vi "Hide not selected Sub-Ctls.vi"(6 "sub":T1[](array[typedef]), 8 "error in":errorcluster, 9 "Sub-Ctls":refnum<vi>[](array[refnum]), 10 "Sub-Ctl Visible":refnum<vi>, 11 "VBox Layout":refnum<class "HSE VBoxLayout.lvclass">) -> (0 "error out":errorcluster, 3 "VBox Layout":refnum<class "HSE VBoxLayout.lvclass">)   [LabVIEW 2022 SP3, in "Navigation.lvlib"]
doc: "____\nHAMPEL SOFTWARE ENGINEERING v2.6.0 (2023-12-19 10:54)"
uses:
  Navigation.lvlib
  <vilib>/Hampel Software Engineering/HSE Layout Manager/HSE Layout/HSE VBoxLayout/HSE VBoxLayout.lvclass
  Button Manager/Sub Control.ctl
  Button Manager/Button Manager.lvclass
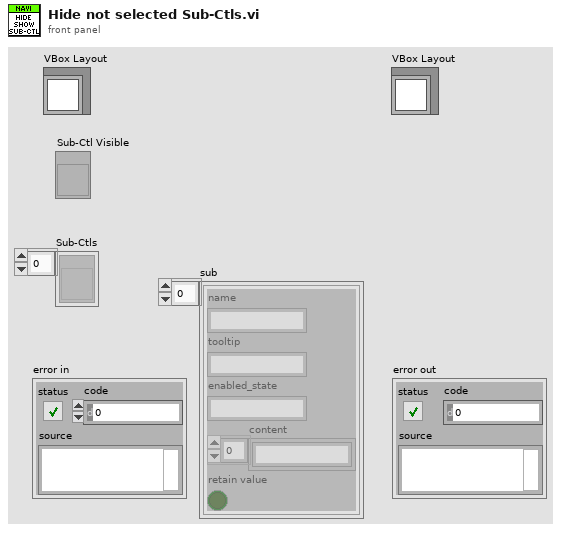
[diagram p1: front panel]
types:
  T1 = typedef "Navigation.lvlib/Button Manager.lvclass/Sub Control.ctl" = cluster{"name":string, "tooltip":string, "enabled_state":string, "content":string[], "retain value":bool}
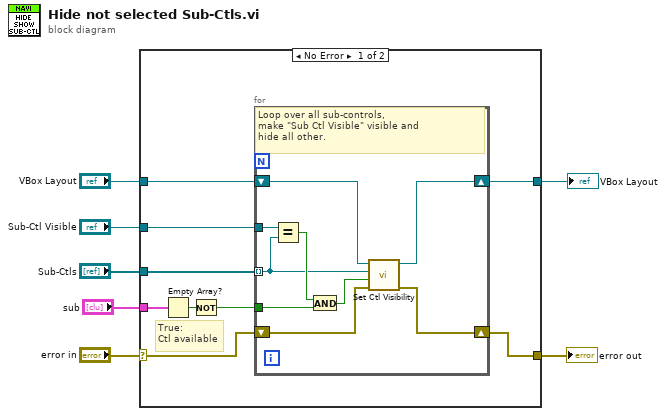
[diagram p0: block diagram]
diagram:
  n1 = case shown="No Error" "error in" {
    selector: "error in" -> [w14 w27]
    tunnel: "Sub-Ctl Visible" -> [w16 _]
    tunnel: "VBox Layout" -> [w15 w26]
    tunnel: [w12 w27] -> w4
    tunnel: "Sub-Ctls" -> [w13 _]
    tunnel: [w11 w26] -> w2
    tunnel: "sub" -> [w10 _]
    frame No Error {
      # "True:\nCtl available"
      n2 = Empty Array?(array=w10) -> (empty?=w9:bool)
      n3 = Not(x=w9) -> (.not. x?=w8:bool)
      n4 = for {
        tunnel: w16 -> [w23]
        tunnel: w13 -> [w17] mode=indexing
        shift-right: [w21] -> w11
        shift-left: w15 -> [w25]
        shift-right: [w20] -> w12
        shift-left: w14 -> [w24]
        tunnel: w8 -> [w18]
        # "Loop over all sub-controls,\nmake \"Sub Ctl Visible\" visible and\nhide all other."
        n5 = Equal?(x=w23, y=w17) -> (x = y?=w22:bool)
        n6 = And(x=w22, y=w18) -> (x .and. y?=w19:bool)
        n7 = call-dynamic "Set Ctl Visibility.vi"("error in"=w24, "Visible?"=w19, "Ctl Refnum"=w17, "HSE Layout in"=w25) -> ("error out"=w20:errorcluster, "HSE Layout out"=w21:refnum<class "HSE VBoxLayout.lvclass">)  [unwired: 5 in, 1 out]
      }
    }
    frame Error {
    }
  }
  "error out" <- w4
  "VBox Layout" <- w2
